vi "OutSettings1.vi"(8 "串口电流计模拟":string[](array[string]), 9 "执行:调用时显示前面板":bool, 10 "电流源输出开关":T1(ring), 11 "电压脉冲卡选择":string[](array[string])) -> (0 "串口电流服务选定口":string[](array[string]), 1 "电流输出开/关":bool, 2 "电压脉冲开关 2":bool, 3 "电压脉冲卡选":u16, 4 "波特率set":u32, 5 "模拟探测器电流源输出 2":bool)   [LabVIEW 2020]
panel:
  in  "模拟探测器电流源输出":bool
  in  "串口电流值服务2":u16(ring)
  out "面板开":bool
  in  "波特率":u32=57600
  in  "串口电流值服务1":u16(ring)
  in  "KEITHLEY622X电流输出开关":bool
  in  "电压脉冲开关":bool
  in  "电压脉冲卡选择":u16(ring)
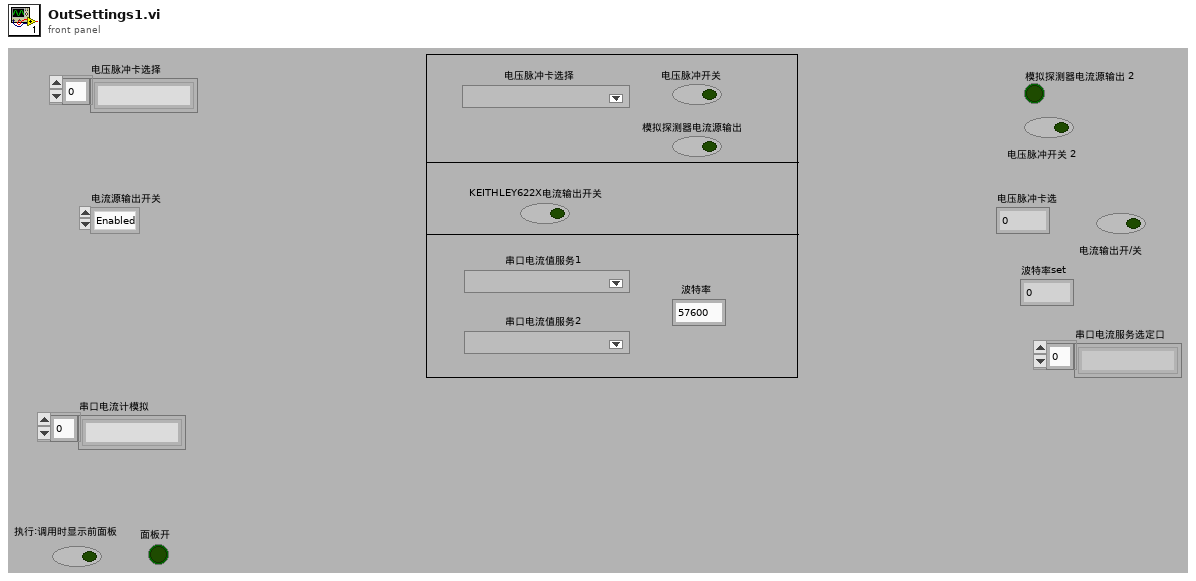
[diagram p1: front panel]
types:
  T1 = enum8{"Enabled", "Disabled", "Disabled and Grayed Out"}
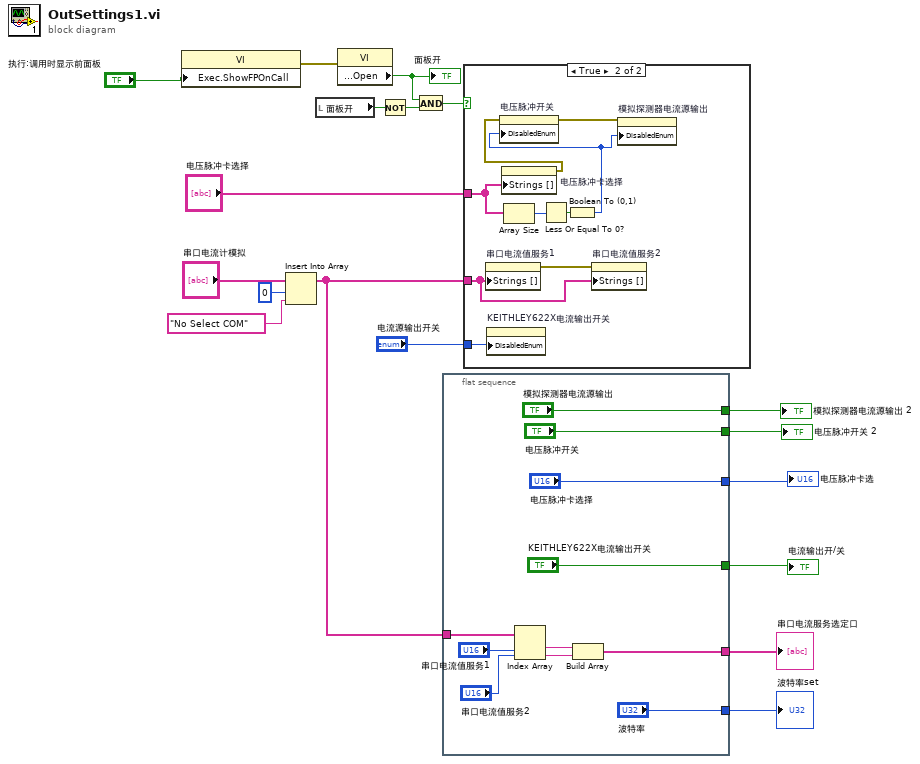
[diagram p0: block diagram]
diagram:
  n1 = property class="VI"("Exec.ShowFPOnCall"="执行:调用时显示前面板") -> (error out=w15:errorcluster)  [unwired: 2 in, 1 out]
  n2 = Insert Into Array(array="串口电流计模拟", index=0 ("索引"), new element="No Select COM" ("新元素/子数组")) -> (w4:string[])
  n3 = local read "面板开"() -> (w14:bool)
  n4 = property class="VI"(error in=w15) -> ("Front Panel.Open"=w12:bool)  [unwired: 1 in, 2 out]
  "面板开" <- w12
  n5 = Not(x=w14) -> (.not. x?=w13:bool)
  n6 = And(x=w12, y=w13) -> (x .and. y?=w11:bool)
  n7 = flat-sequence {
    tunnel: ["电压脉冲开关"] -> w18
    tunnel: ["KEITHLEY622X电流输出开关"] -> w17
    tunnel: ["波特率"] -> w5
    tunnel: w4 -> [w26]
    tunnel: [w21] -> w9
    tunnel: ["电压脉冲卡选择"] -> w2
    tunnel: ["模拟探测器电流源输出"] -> w1
    frame #0 {
      n8 = Index Array(array=w26, index #1="串口电流值服务1", index #2="串口电流值服务2") -> (element #1=w23:string, element #2=w22:string)
      n9 = Build Array(w23, w22) -> (w21:string[])
    }
  }
  n10 = case shown="True" w11 {
    tunnel: "电压脉冲卡选择" -> [_ w36]
    tunnel: w4 -> [_ w34]
    tunnel: "电流源输出开关" -> [_ w35]
    frame False {
    }
    frame True {
      n11 = property on="串口电流值服务1" class="Ring (strict)"("Strings []"=w34) -> (error out=w33:errorcluster)  [unwired: 2 in, 1 out]
      n12 = property on="KEITHLEY622X电流输出开关" class="Bool (strict)"("DisabledEnum"=w35) -> ()  [unwired: 2 in, 2 out]
      n13 = property on="电压脉冲卡选择" class="Ring (strict)"("Strings []"=w36) -> (error out=w32:errorcluster)  [unwired: 2 in, 1 out]
      n14 = Array Size(array=w36) -> (size(s)=w38:i32)
      n15 = Less Or Equal To 0?(x=w38) -> (x <= 0?=w37:bool)
      n16 = Boolean To (0,1)(Boolean=w37) -> (0, 1=w30:i16)
      n17 = property on="电压脉冲开关" class="Bool (strict)"(error in=w32, "DisabledEnum"=w30) -> (error out=w31:errorcluster)  [unwired: 1 in, 1 out]
      n18 = property on="串口电流值服务2" class="Ring (strict)"(error in=w33, "Strings []"=w34) -> ()  [unwired: 1 in, 2 out]
      n19 = property on="模拟探测器电流源输出" class="Bool (strict)"(error in=w31, "DisabledEnum"=w30) -> ()  [unwired: 1 in, 2 out]
    }
  }
  "电压脉冲开关 2" <- w18
  "电流输出开/关" <- w17
  "串口电流服务选定口" <- w9
  "波特率set" <- w5
  "电压脉冲卡选" <- w2
  "模拟探测器电流源输出 2" <- w1
